vi "GlobalVar.vi"(8 "Type Definition":enum16{"Set", "Get"}(ring), 11 "Param in":T3={"sound format"={"sample rate (S/s)"=22050.0, "number of channels"=2, "bits per sample"=16}, "number of samples/ch"=100000, "Play Button"=FALSE, "Device"=0.0, "sample mode"=1} {"sample mode" items=["Finite Samples", "Continuous Samples"]}) -> (3 "Param out":T3 {"sample mode" items=["Finite Samples", "Continuous Samples"]})   [LabVIEW 2015]
uses:
  <vilib>/sound2/lvsound2.llb/Sound Data Format.ctl
  <vilib>/sound2/lvsound2.llb/Sampling Mode.ctl
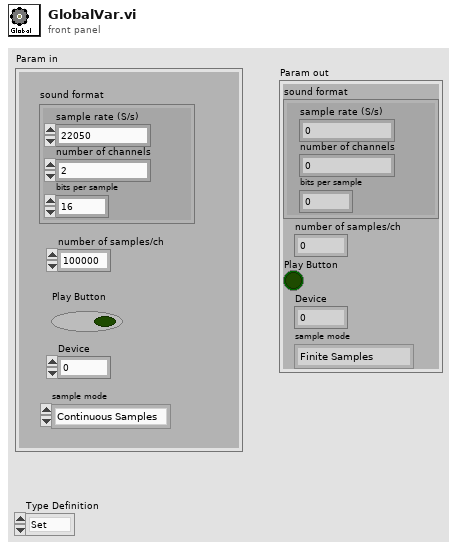
[diagram p1: front panel]
types:
  T1 = typedef "Sound Data Format.ctl" = cluster{"sample rate (S/s)":dbl, "number of channels":i32, "bits per sample":i32}
  T2 = typedef "Sampling Mode.ctl" = i32
  T3 = cluster{"sound format":T1, "number of samples/ch":i32, "Play Button":bool, "Device":dbl, "sample mode":T2}
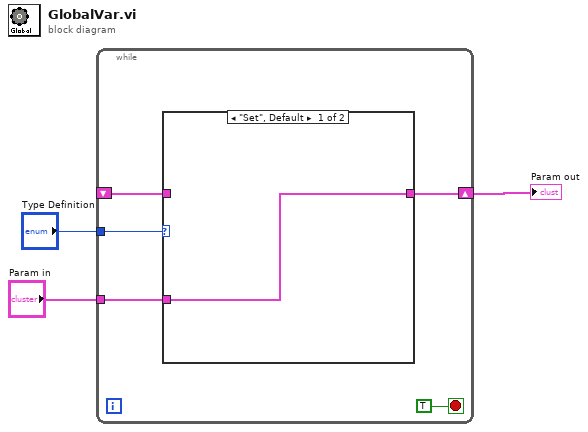
[diagram p0: block diagram]
diagram:
  n1 = while {
    tunnel: "Param in" -> [w6]
    shift-right: [w7] -> w1
    shift-left: _ -> [w5]
    tunnel: "Type Definition" -> [w8]
    stop <- TRUE stop-if-true
    n2 = case shown="\"Set\", Default" w8 {
      tunnel: [w9 w10] -> w7
      tunnel: w6 -> [w9 _]
      tunnel: w5 -> [_ w10]
      frame "Set", Default {
      }
      frame "Get" {
      }
    }
  }
  "Param out" <- w1
